vi "Analyzer.vi"() -> ()   [LabVIEW 2021]
uses:
  LabViewZadania/Zmienna_Globalna.vi
  <vilib>/measure/mascope.llb/Cycle Average and RMS 1 chan.vi
  <vilib>/measure/madcrms.llb/Averaged DC-RMS for 1 Chan.vi
  <vilib>/addons/_NISVFA/_Baseband FFT/SVFA FFT Spectrum (Mag-Phase) (1 Ch).vi
  <vilib>/measure/NI_MAPro.lvlib
panel:
  out "Magnitude":cluster{"f0":dbl, "df":dbl, "magnitude":dbl[]}(graph)
  out "phase":cluster{"f0":dbl, "df":dbl, "phase":dbl[]}(graph)
  out "RMS":dbl format="%0.2f"
  out "Average DC":dbl format="%0.2f"
  out "Sygnal":waveform(dbl)(graph)
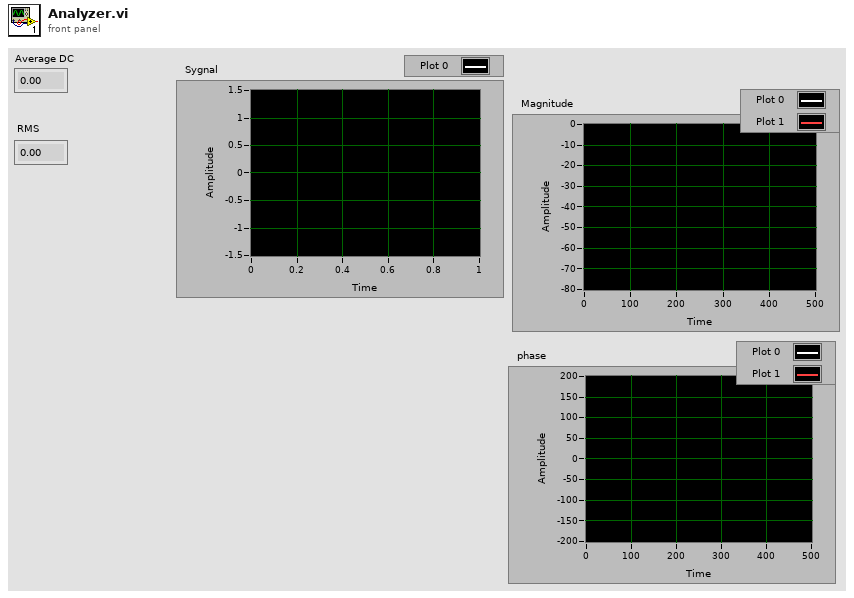
[diagram p1: front panel]
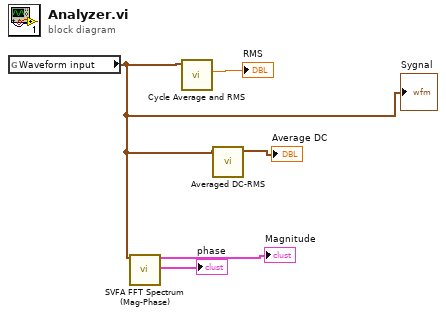
[diagram p0: block diagram]
diagram:
  n1 = global read "Zmienna_Globalna.vi" "Waveform input"() -> (w1:waveform(dbl))
  "Sygnal" <- w1
  n2 = call-poly <vilib>:"SVFA FFT Spectrum (Mag-Phase).vi"("scaled signal [EU]"=w1) -> ("magnitude [dB EU]"=→"Magnitude":cluster{"f0":dbl, "df":dbl, "magnitude":dbl[]}, "phase [degrees]"=→"phase":cluster{"f0":dbl, "df":dbl, "phase":dbl[]})  [unwired: 11 in, 6 out]
  n3 = call-poly <vilib>:"Cycle Average and RMS.vi"("signal in"=w1) -> ("cycle RMS"=→"RMS":dbl)  [unwired: 7 in, 3 out]
  n4 = call-poly <vilib>:"Averaged DC-RMS.vi"("signal in"=w1) -> ("DC value waveform"=→"Average DC":waveform(dbl))  [unwired: 6 in, 4 out]
